vi "HOST.vi"() -> ()   [LabVIEW 2018]
uses:
  <vilib>/userdefined/High Color/nirio_resource_hc.ctl
  <instrlib>/niDCPower/nidcpower.llb/niDCPower Measurement Type.ctl
  <vilib>/FPGAPlugInAG/PXI-7953R/niLvFpga_Open_PXI-7953R.vi
  <vilib>/rvi/interface/common/dynamic/niFpgaDynamicAddResources.vi
  <vilib>/FPGAPlugInAG/Dynamic/niLvFpga_Reset_Dynamic.vi
  <vilib>/FPGAPlugInAG/Dynamic/niLvFpga_Run_Dynamic.vi
  <vilib>/Utility/error.llb/Error Cluster From Error Code.vi
  <vilib>/rvi/errors/niLvFpgaAdjustHostInterfaceError.vi
  <vilib>/rvi/interface/nirviOpenFPGA/nirviOpenFPGA.xnode
  FPGA Bitfiles/ILX751B20.008_FPGATarget_TARGET_7CPBKhOoNyI.lvbitx
  <vilib>/rvi/interface/nirviMethod/nirviMethod.xnode
  <vilib>/rvi/interface/nirviReadWriteControl/nirviReadWriteControl.xnode
  NiFpgaLv.dll
  <vilib>/rvi/interface/Simulation/niFpgaSimulationCallBeginRW.vi
  <vilib>/FPGAPlugInAG/Dynamic/niLvFpga_ReadFifo_Dynamic.vi
  <vilib>/rvi/errors/niLvFpgaMergeErrorWithErrorCode.vi
panel:
  in  "Какой шум на других каналах, мВ?":dbl
  in  "Кадр виден?":u32=50
  in  "3":refnum<k15>="PXI1Slot4" caption="1"
  in  "8191?":u16=8191
  out "DSNU, мВ":dbl
  out "PRNU, %":dbl
  out "|Vout|, мВ":dbl
  in  "Задержка, мкс":u16=7904
  in  "50?":u16=50
  in  "Светлый (T)\nТемный (F)":bool
  in  "Frames":path=path "C:/VPL/LabView_PRJ/ILX751B_20.008/FRAMES"
  in  "ПРИМЕЧАНИЕ":string
  out "Image":T1(plugin-control)
  out "Тнак, мс":dbl=10.0
  in  "Запись в FIFO":bool
  out "АЦП прошит!":bool
  in  "Какой канал?":enum16{"GREEN", "RED", "BLUE"}(ring)=enum."BLUE"
  in  "Усиление (до 6)_RED":u8=1
  in  "Усиление (до 6)_BLUE":u8=1
  in  "Усиление (до 6)_GREEN":u8=1
  in  "Смещение, до 300_BLUE":dbl
  in  "+/- BLUE":enum16{"-", "+"}(ring)=enum."+"
  in  "Смещение, до 300_RED":dbl
  in  "+/- RED":enum16{"-", "+"}(ring)=enum."+"
  in  "Смещение, до 300_GREEN":dbl
  in  "+/- GREEN":enum16{"-", "+"}(ring)=enum."+"
  in  "2/4 V":enum16{"2V", "4V"}(ring)=enum."4V"
  in  "3CH/1CH":enum16{"3CH", "1CH"}(ring)=enum."1CH"
  out "Configuration":bool[](array[boolean])
  in  "HIGH":u8=18
  in  "LOW":u8=8
  in  "CLK_1":u16=59
  in  "ROG_1":u16=20
  in  "ROG_2":u16=40
  in  "SHUT1":u16=120
  in  "CLK_2":u8=9
  in  "CLK_3":u8=20
  in  "20":u8=20
  in  "42000?":u16=42000
  in  "П_41789?":u16=41789
  in  "ADC_2":u8=13
  in  "ADC_1":u8=2
  in  "CDS2_2":u8=16
  in  "CDS2_1":u8=11
  in  "CDS1_2":u8=7
  in  "CDS1_1":u8=2
  in  "Линейки":bool
  in  "Направление бит":bool
  out "VDD2(5)":bool
  out "D_POW":bool
  out "VDD1(9)":bool
  out "A_POW":bool
  in  "VDD2(5)_selcur":dbl=0.019999999999999997 caption="current limit" format="%_6p"
  in  "D_POW_selcur":dbl=0.095 caption="current limit" format="%_6p"
  in  "VDD1(9)_selcur":dbl=0.02 caption="current limit" format="%_6p"
  in  "A_POW_selcur":dbl=0.095 caption="current limit" format="%_6p"
  out "VDD2(5)_char":dbl(graph)=-2.7174410869378702e-06
  out "D_POW_char":dbl(graph)=3.6139019911277516e-06
  in  "VDD2(5), V":dbl=5.0 caption="voltage level" format="%_6p"
  out "VDD2(5)_cur":dbl caption="measurement" format="%_6g"
  out "D_POW_cur":dbl caption="measurement" format="%_6g"
  in  "VDD2(5)_curlim":dbl=0.03 caption="current limit" format="%_6p"
  in  "D_POW_curlim":dbl=0.1 caption="current limit" format="%_6p"
  in  "D_POW, V":dbl=6.0 caption="voltage level" format="%_6p"
  out "VDD1(9)_char":dbl(graph)=-2.1008668383050173e-06
  out "A_POW_char":dbl(graph)=-8.364806008166422e-06
  in  "VDD1(9), V":dbl=9.0 caption="voltage level" format="%_6p"
  out "VDD1(9)_cur":dbl caption="measurement" format="%_6g"
  out "A_POW_cur":dbl caption="measurement" format="%_6g"
  in  "VDD1(9)_curlim":dbl=0.025 caption="current limit" format="%_6p"
  in  "A_POW_curlim":dbl=0.1 caption="current limit" format="%_6p"
  in  "A_POW, V":dbl=6.0 caption="voltage level" format="%_6p"
  in  "Запись кадра":bool
  in  "Прошить АЦП":bool
  in  "Стоп":bool
  in  "Питание":bool
  in  "1":refnum<k15>="PXI1Slot2"
  in  "2":refnum<k15>="PXI1Slot3" caption="1"
  in  "FPGA":T2="PXI1Slot6"
  in  "LOGS":path=path "C:/VPL/LabView_PRJ/ILX751B_20.008/LOGS"
  out "Номер образца":string="0"
  out "Температура":string="0"
  out "DATA":u16[][](array[numeric])=[[50262, 50314, 50369, 50314, 50358, 50311, 50219, 50342, 50335, 50313, 50333, 50279, 50363, 50343, 50274, 50276, 50233, 50283, 50311, 50287, 50326, 50286, 50307, 50313, 50307, 50331, 50315, 50337, 50306, 50335, 50319, 50301, 50336, 50227, 50277, 50229], [50350, 50364, 50285, 50278, 50292, 50197, 50322, 50306, 50283, 50316, 50366, 50335, 50361, 50305, 50282, 50331, 50289, 50304, 50280, 50343, 50359, 50302, 50322, 50214, 50283, 50259, 50363, 50351, 50343, 50321, 50257, 50285, 50351, 50343, 50338, 50332], [50366, 50361, 50275, 50313, 50304, 50293, 50288, 50317, 50370, 50362, 50234, 50266, 50286, 50291, 50335, 50393, 50273, 50357, 50309, 50337, 50280, 50288, 50318, 50296, 50332, 50300, 50286, 50237, 50266, 50342, 50300, 50253, 50340, 50319, 50339, 50302], [50354, 50256, 50301, 50345, 50299, 50339, 50302, 50346, 50308, 50371, 50355, 50325, 50269, 50290, 50285, 50295, 50330, 50336, 50273, 50328, 50381, 50309, 50322, 50368, 50264, 50312, 50320, 50313, 50312, 50334, 50268, 50322, 50334, 50286, 50261, 50358], [50287, 50325, 50343, 50290, 50297, 50249, 50310, 50231, 50393, 50382, 50314, 50281, 50335, 50394, 50319, 50265, 50294, 50289, 50347, 50253, 50336, 50295, 50322, 50299, 50378, 50258, 50375, 50333, 50303, 50337, 50319, 50319, 50298, 50267, 50314, 50295], [50353, 50353, 50335, 50237, 50317, 50296, 50234, 50359, 50320, 50320, 50278, 50331, 50287, 50292, 50318, 50341, 50385, 50311, 50376, 50379, 50338, 50414, 50297, 50260, 50227, 50299, 50319, 50396, 50380, 50305, 50335, 50281, 50362, 50368, 50336, 50293], [50306, 50281, 50350, 50290, 50282, 50309, 50310, 50345, 50257, 50309, 50334, 50377, 50244, 50252, 50260, 50349, 50408, 50298, 50304, 50320, 50314, 50316, 50265, 50294, 50400, 50263, 50304, 50272, 50319, 50392, 50327, 50280, 50360, 50255, 50358, 50361], [50350, 50246, 50307, 50293, 50282, 50315, 50263, 50291, 50402, 50315, 50351, 50325, 50369, 50243, 50347, 50363, 50304, 50328, 50247, 50311, 50333, 50430, 50262, 50343, 50369, 50284, 50307, 50319, 50305, 50258, 50334, 50339, 50319, 50380, 50365, 50363], [50349, 50329, 50280, 50304, 50335, 50280, 50314, 50306, 50298, 50357, 50316, 50381, 50295, 50289, 50218, 50298, 50346, 50225, 50386, 50297, 50333, 50311, 50310, 50235, 50280, 50290, 50309, 50275, 50289, 50386, 50273, 50300, 50357, 50360, 50305, 50350], [50332, 50310, 50312, 50284, 50303, 50332, 50307, 50290, 50276, 50337, 50376, 50371, 50329, 50360, 50328, 50316, 50329, 50346, 50292, 50326, 50338, 50284, 50331, 50256, 50333, 50351, 50274, 50375, 50312, 50302, 50347, 50301, 50341, 50276, 50235, 50295], [50368, 50274, 50286, 50317, 50311, 50276, 50267, 50303, 50282, 50301, 50318, 50259, 50361, 50309, 50320, 50255, 50223, 50330, 50380, 50312, 50369, 50261, 50323, 50266, 50374, 50210, 50374, 50289, 50329, 50331, 50301, 50281, 50270, 50310, 50367, 50268], [50304, 50349, 50357, 50309, 50320, 50276, 50360, 50358, 50320, 50316, 50280, 50238, 50371, 50312, 50236, 50334, 50295, 50391, 50334, 50300, 50341, 50353, 50305, 50233, 50234, 50266, 50322, 50294, 50306, 50397, 50267, 50307, 50365, 50369, 50336, 50331], [50309, 50374, 50308, 50336, 50307, 50284, 50361, 50352, 50378, 50343, 50340, 50308, 50268, 50279, 50363, 50340, 50314, 50294, 50299, 50325, 50276, 50301, 50383, 50309, 50320, 50314, 50266, 50391, 50338, 50232, 50405, 50285, 50299, 50281, 50352, 50288], [50324, 50243, 50342, 50322, 50352, 50352, 50305, 50253, 50309, 50250, 50270, 50266, 50292, 50292, 50351, 50309, 50317, 50312, 50360, 50335, 50310, 50304, 50262, 50340, 50305, 50309, 50320, 50321, 50328, 50282, 50334, 50304, 50300, 50320, 50305, 50313], [50326, 50354, 50306, 50316, 50338, 50313, 50369, 50327, 50318, 50357, 50354, 50312, 50363, 50327, 50338, 50381, 50312, 50319, 50261, 50309, 50318, 50354, 50349, 50340, 50356, 50325, 50291, 50232, 50350, 50346, 50276, 50383, 50290, 50281, 50281, 50342], [50361, 50273, 50328, 50306, 50307, 50246, 50290, 50388, 50343, 50389, 50305, 50283, 50336, 50403, 50288, 50346, 50371, 50282, 50355, 50334, 50297, 50351, 50387, 50371, 50289, 50292, 50321, 50269, 50295, 50356, 50238, 50360, 50346, 50359, 50314, 50301], [50252, 50301, 50331, 50337, 50242, 50286, 50276, 50311, 50302, 50325, 50333, 50308, 50329, 50327, 50344, 50354, 50316, 50272, 50257, 50354, 50361, 50344, 50372, 50284, 50301, 50326, 50348, 50334, 50366, 50302, 50291, 50302, 50285, 50349, 50279, 50285], [50295, 50324, 50312, 50371, 50300, 50301, 50322, 50338, 50385, 50358, 50374, 50369, 50315, 50364, 50239, 50389, 50322, 50323, 50272, 50333, 50322, 50343, 50313, 50268, 50362, 50359, 50315, 50302, 50358, 50329, 50299, 50295, 50263, 50367, 50354, 50277], [50285, 50253, 50337, 50323, 50334, 50348, 50350, 50292, 50307, 50305, 50262, 50413, 50304, 50307, 50286, 50313, 50318, 50406, 50369, 50319, 50306, 50385, 50329, 50396, 50247, 50377, 50372, 50334, 50322, 50381, 50364, 50304, 50325, 50317, 50330, 50190], [50336, 50338, 50322, 50295, 50419, 50350, 50295, 50371, 50329, 50321, 50293, 50299, 50347, 50374, 50348, 50310, 50349, 50397, 50395, 50242, 50273, 50312, 50298, 50291, 50343, 50312, 50338, 50295, 50327, 50323, 50416, 50285, 50281, 50289, 50289, 50308], [50348, 50318, 50252, 50326, 50350, 50324, 50311, 50284, 50307, 50361, 50328, 50345, 50294, 50315, 50312, 50390, 50336, 50273, 50349, 50286, 50363, 50346, 50322, 50316, 50335, 50349, 50311, 50275, 50298, 50273, 50344, 50269, 50287, 50349, 50376, 50296], [50346, 50375, 50300, 50310, 50332, 50321, 50281, 50344, 50327, 50344, 50314, 50296, 50264, 50303, 50292, 50249, 50272, 50352, 50341, 50286, 50350, 50288, 50264, 50288, 50339, 50331, 50304, 50306, 50316, 50303, 50273, 50326, 50293, 50312, 50371, 50314], [50323, 50330, 50320, 50367, 50295, 50329, 50297, 50278, 50345, 50341, 50284, 50252, 50343, 50350, 50360, 50332, 50276, 50305, 50345, 50342, 50314, 50376, 50420, 50322, 50313, 50363, 50318, 50338, 50333, 50290, 50335, 50263, 50301, 50286, 50337, 50249], [50343, 50348, 50377, 50338, 50382, 50269, 50308, 50370, 50305, 50383, 50350, 50392, 50367, 50304, 50281, 50327, 50286, 50313, 50308, 50270, 50333, 50319, 50326, 50282, 50395, 50342, 50297, 50331, 50297, 50323, 50275, 50276, 50323, 50278, 50279, 50321], [50230, 50351, 50349, 50291, 50304, 50283, 50315, 50264, 50387, 50292, 50319, 50259, 50376, 50275, 50388, 50293, 50343, 50254, 50299, 50334, 50276, 50381, 50315, 50347, 50303, 50278, 50376, 50293, 50367, 50287, 50311, 50340, 50288, 50319, 50375, 50299], [50304, 50338, 50255, 50333, 50353, 50298, 50321, 50241, 50274, 50296, 50317, 50350, 50284, 50385, 50270, 50276, 50349, 50228, 50340, 50267, 50376, 50352, 50328, 50286, 50267, 50386, 50324, 50342, 50331, 50339, 50331, 50346, 50355, 50319, 50271, 50291], [50315, 50259, 50331, 50329, 50311, 50329, 50347, 50403, 50324, 50381, 50316, 50273, 50285, 50338, 50298, 50312, 50326, 50298, 50307, 50387, 50362, 50315, 50299, 50383, 50327, 50393, 50323, 50285, 50357, 50387, 50270, 50325, 50308, 50338, 50231, 50285], [50384, 50350, 50363, 50391, 50340, 50290, 50319, 50355, 50291, 50418, 50347, 50265, 50239, 50265, 50343, 50343, 50400, 50315, 50292, 50367, 50345, 50326, 50293, 50318, 50345, 50256, 50297, 50262, 50363, 50380, 50330, 50346, 50331, 50429, 50274, 50273], [50329, 50359, 50330, 50399, 50308, 50368, 50289, 50321, 50333, 50340, 50276, 50410, 50324, 50324, 50356, 50370, 50327, 50278, 50340, 50392, 50355, 50329, 50375, 50282, 50324, 50353, 50288, 50345, 50281, 50350, 50254, 50322, 50266, 50288, 50267, 50287], [50397, 50341, 50356, 50357, 50321, 50300, 50278, 50294, 50284, 50374, 50242, 50349, 50325, 50326, 50243, 50309, 50404, 50316, 50279, 50313, 50314, 50334, 50274, 50285, 50328, 50315, 50279, 50271, 50340, 50340, 50287, 50351, 50355, 50322, 50284, 50339], [50345, 50387, 50385, 50288, 50353, 50322, 50341, 50374, 50340, 50316, 50369, 50362, 50341, 50276, 50336, 50288, 50347, 50316, 50340, 50258, 50320, 50319, 50292, 50392, 50381, 50374, 50329, 50280, 50310, 50356, 50373, 50386, 50344, 50265, 50250, 50334], [50321, 50238, 50340, 50279, 50339, 50338, 50323, 50336, 50357, 50311, 50365, 50345, 50274, 50350, 50395, 50322, 50330, 50347, 50291, 50291, 50299, 50361, 50255, 50331, 50301, 50305, 50274, 50297, 50363, 50392, 50252, 50391, 50286, 50387, 50278, 50300], [50217, 50371, 50307, 50339, 50290, 50314, 50315, 50337, 50319, 50307, 50239, 50341, 50350, 50283, 50349, 50361, 50338, 50295, 50305, 50344, 50318, 50265, 50273, 50350, 50284, 50361, 50226, 50334, 50331, 50316, 50314, 50319, 50297, 50261, 50266, 50315], [50279, 50360, 50294, 50297, 50343, 50325, 50286, 50335, 50258, 50295, 50374, 50267, 50359, 50313, 50265, 50281, 50287, 50343, 50338, 50356, 50330, 50309, 50297, 50345, 50330, 50329, 50320, 50320, 50340, 50311, 50264, 50258, 50334, 50294, 50287, 50320], [50297, 50313, 50389, 50289, 50356, 50348, 50342, 50368, 50390, 50300, 50328, 50251, 50290, 50217, 50338, 50416, 50363, 50333, 50326, 50301, 50270, 50301, 50264, 50365, 50290, 50299, 50302, 50326, 50304, 50303, 50289, 50269, 50319, 50290, 50293, 50322], [50294, 50349, 50301, 50344, 50301, 50333, 50344, 50296, 50326, 50380, 50368, 50268, 50284, 50287, 50296, 50302, 50336, 50278, 50299, 50352, 50311, 50302, 50275, 50315, 50360, 50293, 50355, 50299, 50323, 50298, 50356, 50279, 50343, 50337, 50251, 50336], [50247, 50377, 50328, 50357, 50314, 50287, 50326, 50310, 50324, 50323, 50325, 50313, 50327, 50304, 50329, 50250, 50348, 50455, 50386, 50310, 50383, 50312, 50349, 50233, 50295, 50397, 50284, 50320, 50260, 50291, 50328, 50278, 50336, 50262, 50259, 50306], [50359, 50342, 50327, 50305, 50335, 50317, 50367, 50285, 50340, 50357, 50344, 50287, 50346, 50348, 50290, 50304, 50343, 50297, 50328, 50381, 50298, 50265, 50406, 50262, 50350, 50269, 50206, 50385, 50325, 50265, 50298, 50293, 50374, 50284, 50352, 50335], [50342, 50353, 50288, 50360, 50419, 50337, 50312, 50326, 50324, 50359, 50356, 50300, 50215, 50284, 50335, 50312, 50328, 50287, 50316, 50281, 50298, 50302, 50289, 50322, 50368, 50289, 50333, 50250, 50291, 50346, 50270, 50304, 50321, 50363, 50343, 50331], [50352, 50280, 50263, 50251, 50331, 50290, 50298, 50329, 50399, 50351, 50337, 50287, 50304, 50329, 50381, 50376, 50343, 50284, 50320, 50242, 50308, 50273, 50288, 50316, 50379, 50336, 50260, 50350, 50378, 50349, 50290, 50334, 50275, 50291, 50376, 50283], [50377, 50367, 50281, 50214, 50311, 50318, 50299, 50270, 50249, 50259, 50321, 50371, 50315, 50290, 50285, 50286, 50255, 50359, 50385, 50386, 50221, 50283, 50329, 50352, 50261, 50308, 50291, 50272, 50294, 50354, 50296, 50299, 50288, 50297, 50275, 50292], [50321, 50326, 50282, 50349, 50268, 50298, 50309, 50365, 50344, 50278, 50341, 50362, 50340, 50230, 50289, 50230, 50327, 50354, 50325, 50358, 50403, 50299, 50351, 50286, 50269, 50319, 50317, 50279, 50235, 50254, 50369, 50348, 50367, 50341, 50277, 50288], [50332, 50357, 50278, 50248, 50312, 50294, 50258, 50305, 50374, 50310, 50361, 50311, 50304, 50341, 50247, 50336, 50337, 50320, 50350, 50351, 50310, 50320, 50258, 50287, 50285, 50347, 50402, 50355, 50293, 50294, 50303, 50367, 50295, 50294, 50329, 50303], [50279, 50371, 50307, 50324, 50277, 50281, 50353, 50317, 50318, 50254, 50314, 50422, 50282, 50269, 50277, 50303, 50355, 50297, 50286, 50318, 50297, 50311, 50370, 50221, 50315, 50356, 50313, 50309, 50254, 50291, 50308, 50240, 50252, 50371, 50403, 50380], [50296, 50318, 50429, 50315, 50282, 50342, 50311, 50282, 50247, 50303, 50323, 50329, 50299, 50389, 50305, 50253, 50294, 50473, 50292, 50316, 50336, 50411, 50408, 50318, 50254, 50356, 50375, 50344, 50355, 50207, 50306, 50327, 50346, 50289, 50303, 50265], [50363, 50305, 50264, 50319, 50350, 50281, 50322, 50336, 50355, 50293, 50298, 50335, 50306, 50329, 50272, 50319, 50333, 50251, 50390, 50284, 50327, 50276, 50301, 50321, 50338, 50295, 50352, 50354, 50386, 50361, 50257, 50276, 50313, 50327, 50352, 50264], [50260, 50306, 50291, 50288, 50350, 50326, 50331, 50273, 50306, 50313, 50309, 50301, 50326, 50347, 50302, 50382, 50372, 50269, 50347, 50289, 50299, 50366, 50324, 50345, 50344, 50295, 50287, 50270, 50352, 50300, 50271, 50301, 50287, 50360, 50264, 50345], [50316, 50327, 50336, 50252, 50314, 50342, 50357, 50370, 50330, 50245, 50305, 50260, 50349, 50353, 50288, 50296, 50286, 50282, 50276, 50284, 50358, 50245, 50323, 50312, 50298, 50303, 50334, 50301, 50338, 50359, 50379, 50299, 50300, 50325, 50343, 50263], [50287, 50306, 50332, 50297, 50215, 50337, 50371, 50298, 50288, 50337, 50324, 50279, 50309, 50296, 50254, 50354, 50333, 50334, 50284, 50405, 50367, 50340, 50281, 50342, 50380, 50341, 50346, 50278, 50261, 50274, 50358, 50281, 50385, 50296, 50275, 50327], [50314, 50340, 50342, 50367, 50309, 50319, 50338, 50379, 50283, 50366, 50347, 50367, 50387, 50229, 50327, 50299, 50243, 50327, 50328, 50345, 50309, 50365, 50321, 50308, 50294, 50306, 50234, 50310, 50306, 50305, 50351, 50403, 50319, 50279, 50270, 50321], [50295, 50311, 50369, 50283, 50256, 50277, 50329, 50350, 50267, 50314, 50384, 50340, 50413, 50363, 50295, 50252, 50246, 50358, 50337, 50355, 50258, 50313, 50327, 50298, 50319, 50399, 50312, 50391, 50305, 50321, 50301, 50336, 50309, 50312, 50300, 50356], [50376, 50314, 50302, 50290, 50314, 50346, 50351, 50319, 50271, 50279, 50305, 50351, 50281, 50363, 50385, 50350, 50357, 50318, 50279, 50330, 50307, 50314, 50335, 50329, 50345, 50317, 50295, 50371, 50258, 50330, 50374, 50239, 50353, 50387, 50329, 50325], [50285, 50280, 50265, 50316, 50314, 50264, 50258, 50262, 50350, 50381, 50336, 50281, 50345, 50305, 50252, 50358, 50318, 50314, 50340, 50334, 50265, 50331, 50305, 50394, 50319, 50374, 50381, 50286, 50349, 50335, 50353, 50380, 50237, 50324, 50283, 50374], [50318, 50292, 50336, 50265, 50301, 50291, 50300, 50336, 50292, 50308, 50363, 50352, 50284, 50342, 50272, 50349, 50476, 50358, 50261, 50350, 50336, 50400, 50421, 50284, 50345, 50320, 50278, 50344, 50338, 50366, 50272, 50323, 50316, 50339, 50371, 50198], [50359, 50322, 50413, 50297, 50295, 50361, 50233, 50330, 50260, 50259, 50350, 50374, 50293, 50306, 50325, 50331, 50295, 50286, 50277, 50360, 50331, 50405, 50243, 50326, 50320, 50333, 50306, 50367, 50343, 50346, 50294, 50309, 50319, 50361, 50361, 50315], [50312, 50309, 50306, 50336, 50269, 50332, 50258, 50295, 50304, 50366, 50386, 50385, 50215, 50292, 50281, 50355, 50290, 50333, 50282, 50216, 50323, 50287, 50350, 50355, 50338, 50275, 50315, 50353, 50325, 50317, 50307, 50399, 50302, 50370, 50346, 50269], [50239, 50355, 50305, 50347, 50338, 50337, 50257, 50334, 50253, 50315, 50306, 50374, 50387, 50344, 50365, 50329, 50317, 50357, 50332, 50338, 50350, 50308, 50258, 50306, 50291, 50335, 50362, 50323, 50325, 50347, 50293, 50367, 0, 0, 0, 50266], [50265, 50281, 50002, 50308, 50309, 50282, 50304, 50313, 50318, 50294, 50341, 50296, 50342, 50319, 50361, 50354, 50328, 50217, 50303, 50266, 50393, 50366, 50374, 50243, 50307, 50246, 50331, 50271, 50223, 50271, 50323, 50293, 50207, 50289, 50339, 0]]
  # "ПРЕДЛАГАЮ БРАТЬ ЗА НАСЫЩЕНИЕ МАКСИМАЛЬНО ДОСТИЖИМОЕ ЗНАЧЕНИЕ"
  # "7904 и 120"
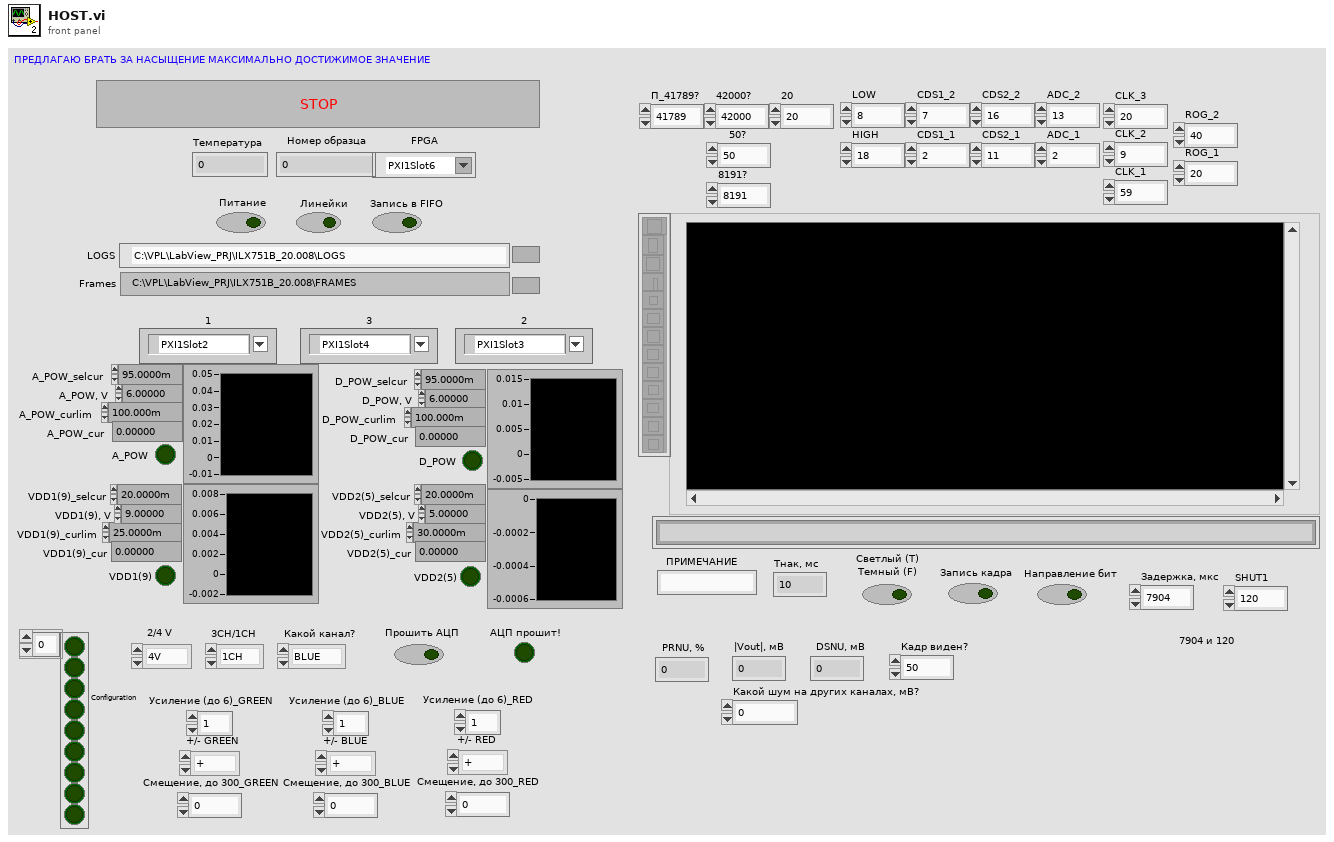
[diagram p1: front panel]
types:
  T1 = typedef "IMAQ Image.ctl" = refnum<image>
  T2 = typedef "nirio_resource_hc.ctl" = tag
  T3 = enum16{"open", "replace", "create", "open or create", "replace or create", "replace or create with confirmation"}
  T4 = enum16{"Configuration", "MUX", "RED PGA", "GREEN PGA", "BLUE PGA", "RED OFF", "GREEN OFF", "BLUE OFF"}
  T5 = typedef "Image Type" = u32
  T6 = typedef "niDCPower Measurement Type.ctl" = i32
  T7 = cluster{"Global Rectangle":i32[], "Contours":cluster{"Contour Type":u32, "ROI Type":u32, "Points":i32[]}[]}
  T8 = cluster{"Contour Type":u32, "ROI Type":u32, "Points":i32[]}[]
  T9 = cluster{"Contour Type":u32, "ROI Type":u32, "Points":i32[]}
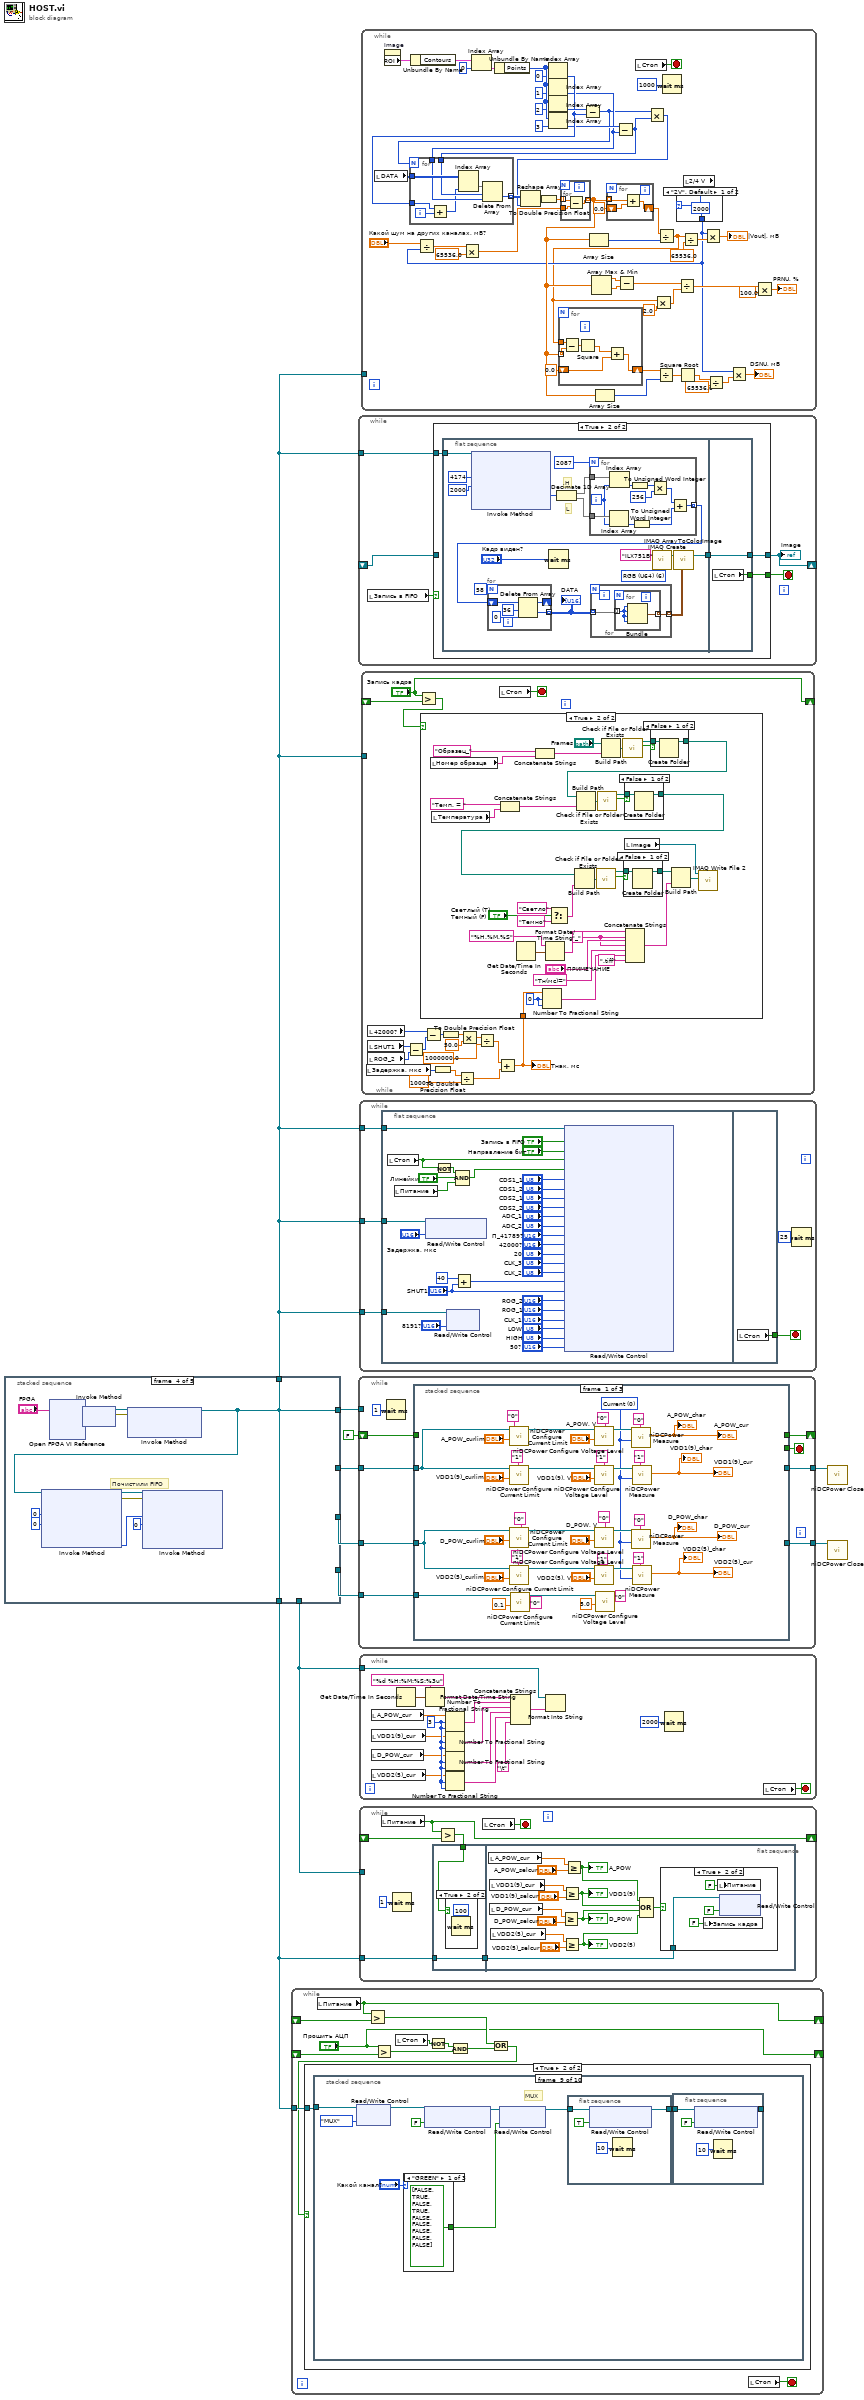
[diagram p0: block diagram]
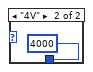
[diagram p2: hidden frame]
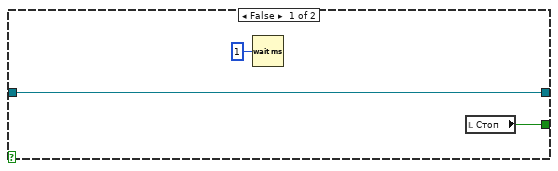
[diagram p3: hidden frame]
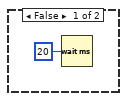
[diagram p4: hidden frame]
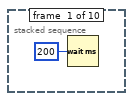
[diagram p5: hidden frame]
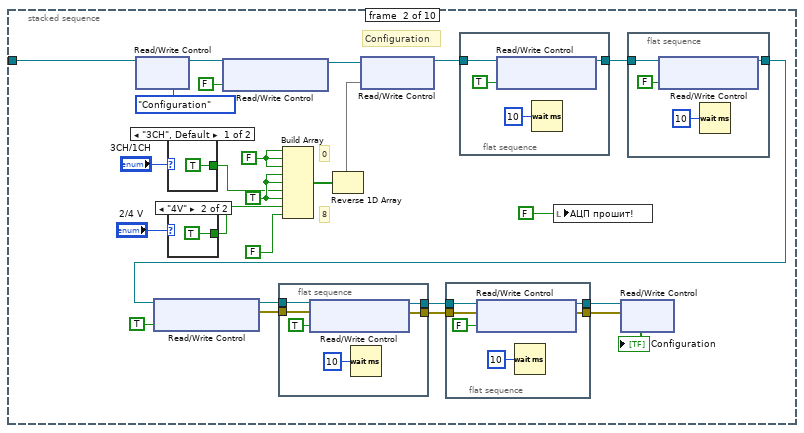
[diagram p6: hidden frame]
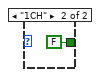
[diagram p7: hidden frame]
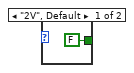
[diagram p8: hidden frame]
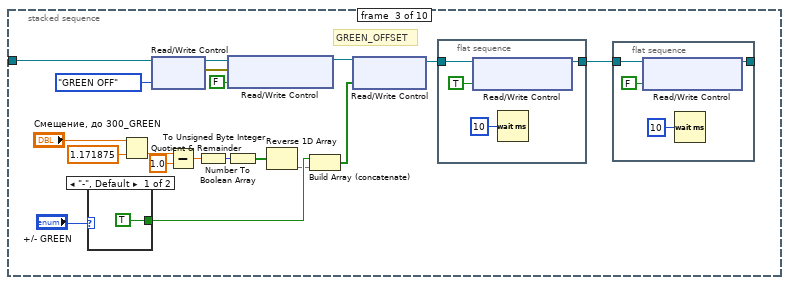
[diagram p9: hidden frame]
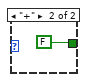
[diagram p10: hidden frame]
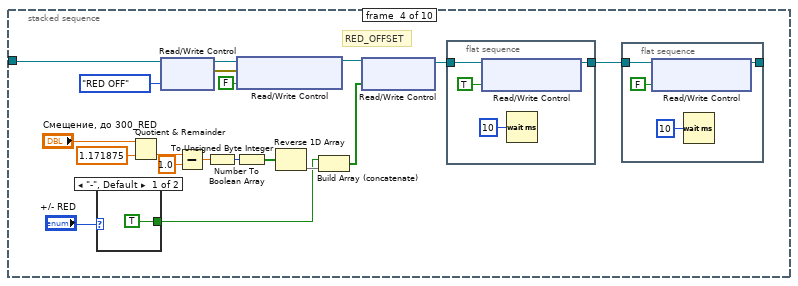
[diagram p11: hidden frame]
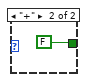
[diagram p12: hidden frame]
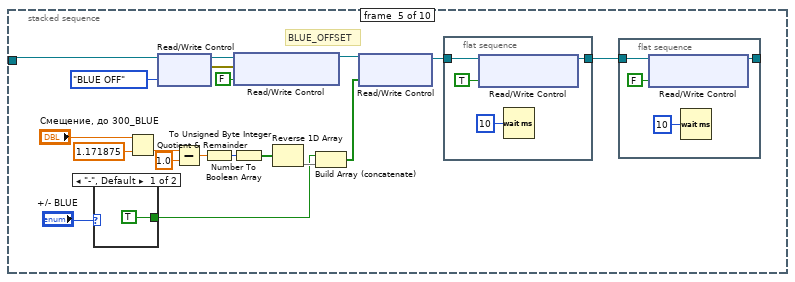
[diagram p13: hidden frame]
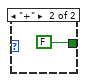
[diagram p14: hidden frame]
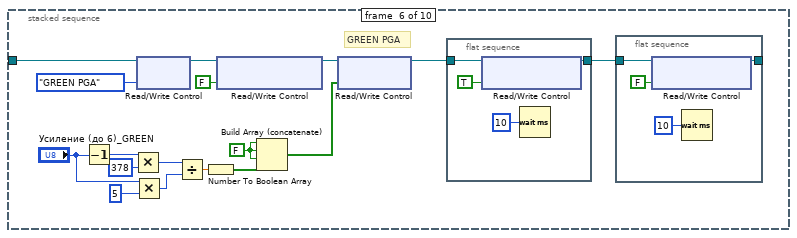
[diagram p15: hidden frame]
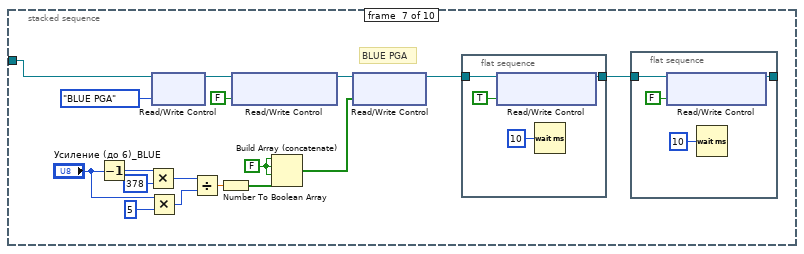
[diagram p16: hidden frame]
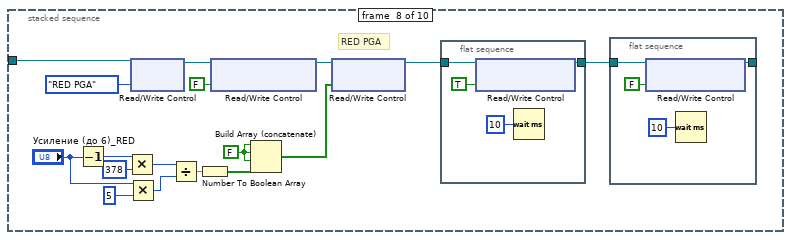
[diagram p17: hidden frame]
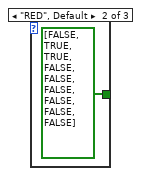
[diagram p18: hidden frame]
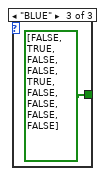
[diagram p19: hidden frame]
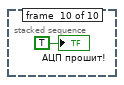
[diagram p20: hidden frame]
diagram:
  n1 = stacked-sequence {
    tunnel: [_ _ _ w61 _] -> w8
    tunnel: [_ _ _ _ w82] -> w10
    tunnel: [_ _ _ _ w81] -> w9
    tunnel: [_ _ _ w61 _] -> w1
    tunnel: [_ _ _ w61 _] -> w3
    tunnel: [_ _ w29 _ _] -> w4
    tunnel: [_ _ _ _ w73] -> w2
    frame #0 {
      n2 = call "Begin.vi"() -> ("Температура 2"=→"Температура":string, "Номер образца 2"=→"Номер образца":string)  [unwired: 10 in]
    }
    frame #1 {
      # "Обнуление всего"
      n3 = local write "Прошить АЦП"(FALSE ("Прошить АЦП")) -> ()
      n4 = local write "Запись кадра"(FALSE ("FRAME!")) -> ()
      n5 = local write "Питание"(FALSE ("Питание")) -> ()
      n6 = local write "Стоп"(FALSE ("Стоп")) -> ()
      n7 = local write "VDD1(9)"(FALSE ("VDD1(9)")) -> ()
      n8 = local write "VDD2(5)"(FALSE ("VDD2(5)")) -> ()
      n9 = local write "A_POW"(FALSE ("A_POW")) -> ()
      n10 = local write "D_POW"(FALSE ("D_POW")) -> ()
    }
    frame #2 {
      w22 = "\t"
      n11 = local read "Номер образца"() -> (w50:string)
      n12 = Build Path(base path="LOGS", name or relative path=w50) -> (appended path=w47:path)
      n13 = Get Date/Time In Seconds() -> (seconds since 1Jan1904=w44:timestamp)
      n14 = call <vilib>:"Check if File or Folder Exists.vi"("path"=w47) -> ("file or folder exists?"=w48:bool, "dup path"=w49:path)  [unwired: 8 in, 1 out]
      n15 = local read "Температура"() -> (w24:string)
      n16 = Format Date/Time String(time format string (%c)="%d %H.%M.%S", seconds (now)=w44) -> (date/time string=w42:string)  [unwired: 1 in]
      n17 = case shown="False" w48 {
        tunnel: w49 -> [w59 w60]
        tunnel: [w58 w60] -> w25
        frame False {
          n18 = Create Folder(path (use dialog)=w59) -> (created path=w58:path)  [unwired: 2 in, 2 out]
        }
        frame True {
        }
      }
      n19 = Concatenate Strings(w42, ".xls" ("string")) -> (w41:string)
      n20 = Build Path(base path=w25, name or relative path=w24) -> (appended path=w28:path)
      n21 = call <vilib>:"Check if File or Folder Exists.vi"("path"=w28) -> ("file or folder exists?"=w27:bool, "dup path"=w26:path)  [unwired: 8 in, 1 out]
      n22 = case shown="False" w27 {
        tunnel: w26 -> [w52 w53]
        tunnel: [w51 w53] -> w23
        frame False {
          n23 = Create Folder(path (use dialog)=w52) -> (created path=w51:path)  [unwired: 2 in, 2 out]
        }
        frame True {
        }
      }
      n24 = Build Path(base path=w23, name or relative path=w41) -> (appended path=w43:path)
      n25 = Open/Create/Replace File(file path (use dialog)=w43, operation (0:open)=T3."open or create", access (0:read/write)=enum16{"read/write", "read-only", "write-only"}."read/write") -> (refnum out=w45:refnum<file>)  [unwired: 3 in, 2 out]
      n26 = case shown="True" TRUE {
        tunnel: w45 -> [w54 w57]
        tunnel: [w54 w55] -> w40
        frame False {
        }
        frame True {
          n27 = Set File Position(refnum=w57, from (0:start)=enum16{"start", "end", "current"}."end") -> (refnum out=w55:refnum<file>)  [unwired: 2 in, 1 out]
        }
      }
      n28 = Format Into String(initial string=w40, "Time" ("input 1"), w22, "A_POW_cur", w22, "VDD1_cur", w22, "D_POW_cur", w22, "VDD2_cur", "\r\n") -> (resulting string=w29:refnum<file>)  [unwired: 2 in, 1 out]
    }
    frame #3 {
      # "Почистили FIFO"
      n29 = xnode "Open FPGA VI Reference"("resource name"="FPGA") -> ("FPGA VI Reference Out"=w69:refnum<k20>, "error out"=w71:errorcluster)  [unwired: 1 in]
      n30 = xnode "Invoke Method"("FPGA VI Reference In"=w69, "error in"=w71) -> ("FPGA VI Reference Out"=w72:refnum<k20>, "error out"=w70:errorcluster)
      n31 = xnode "Invoke Method"("FPGA VI Reference In"=w72, "error in"=w70) -> ("FPGA VI Reference Out"=w61:refnum<k20>)  [unwired: 1 in, 1 out]
      n32 = xnode "Invoke Method"("FPGA VI Reference In"=w61, "Number of Elements"=u32 0, "Timeout (ms)"=0) -> ("FPGA VI Reference Out"=w67:refnum<k20>, "error out"=w66:errorcluster, "Elements Remaining"=w65:u32)  [unwired: 1 in, 1 out]
      n33 = xnode "Invoke Method"("FPGA VI Reference In"=w67, "error in"=w66, "Number of Elements"=w65, "Timeout (ms)"=0) -> ()  [unwired: 4 out]
    }
    frame #4 {
      n34 = call <instrlib>:"niDCPower Initialize.vi"("resource name"="3") -> ("error out"=w76:errorcluster, "instrument handle out"=w77:refnum<k15>)  [unwired: 3 in, 6 out]
      n35 = call <instrlib>:"niDCPower Initialize.vi"("resource name"="2") -> ("error out"=w85:errorcluster, "instrument handle out"=w83:refnum<k15>)  [unwired: 3 in, 6 out]
      n36 = call <instrlib>:"niDCPower Initialize.vi"("resource name"="1") -> ("error out"=w86:errorcluster, "instrument handle out"=w84:refnum<k15>)  [unwired: 3 in, 6 out]
      n37 = call <instrlib>:"niDCPower Configure Voltage Level.vi"("error in (no error)"=w76, "voltage level"=0.0, "channel name"="0", "instrument handle"=w77) -> ("instrument handle out"=w73:refnum<k15>)  [unwired: 6 in, 1 out]
      n38 = call <instrlib>:"niDCPower Configure Voltage Level.vi"("error in (no error)"=w85, "voltage level"=0.0, "channel name"="0,1", "instrument handle"=w83) -> ("instrument handle out"=w81:refnum<k15>)  [unwired: 6 in, 1 out]
      n39 = call <instrlib>:"niDCPower Configure Voltage Level.vi"("error in (no error)"=w86, "voltage level"=0.0, "channel name"="0,1", "instrument handle"=w84) -> ("instrument handle out"=w82:refnum<k15>)  [unwired: 6 in, 1 out]
    }
  }
  n40 = while {
    tunnel: w3 -> [w101]
    shift-right: ["Прошить АЦП"] -> _
    shift-left: _ -> [w100]
    shift-right: [w96] -> _
    shift-left: _ -> [w97]
    stop <- w102 stop-if-true
    n41 = local read "Питание"() -> (w96:bool)
    n42 = Greater?(x=w96, y=w97) -> (0:w95:bool)
    n43 = Greater?(x="Прошить АЦП", y=w100) -> (0:w99:bool)
    n44 = local read "Стоп"() -> (w92:bool)
    n45 = Not(x=w92) -> (.not. x?=w91:bool)
    n46 = And(x=w91, y=w99) -> (x .and. y?=w98:bool)
    n47 = Or(x=w95, y=w98) -> (x .or. y?=w94:bool)
    n48 = case shown="True" w94 {
      tunnel: w101 -> [_ w104]
      frame False {
        n49 = Wait (ms)(milliseconds to wait=u32 20) -> ()  [unwired: 1 out]
      }
      frame True {
        n50 = stacked-sequence {
          tunnel: w104 -> [_ w131 w171 w185 w214 w258 w268 w293 w326 _]
          frame #0 {
            n51 = Wait (ms)(milliseconds to wait=u32 200) -> ()  [unwired: 1 out]
          }
          frame #1 {
            w127 = TRUE ("element")
            w128 = FALSE
            # "8"
            # "0"
            # "Configuration"
            n52 = xnode "Read/Write Control"("FPGA VI Reference In"=w131, "Enum"=T4."Configuration") -> ("FPGA VI Reference Out"=w118:refnum<k20>)  [unwired: 1 in, 1 out]
            n53 = xnode "Read/Write Control"("FPGA VI Reference In"=w108, "Read(T)/Write(F)"=TRUE) -> ("FPGA VI Reference Out"=w114:refnum<k20>, "error out"=w113:errorcluster)  [unwired: 1 in]
            n54 = case shown="\"3CH\", Default" "3CH/1CH" {
              tunnel: [TRUE FALSE] -> w126
              frame "3CH", Default {
              }
              frame "1CH" {
              }
            }
            n55 = case shown="\"4V\"" "2/4 V" {
              tunnel: [FALSE TRUE] -> w124
              frame "2V", Default {
              }
              frame "4V" {
              }
            }
            n56 = xnode "Read/Write Control"("FPGA VI Reference In"=w118, "Read(T)/Write(F)"=FALSE) -> ("FPGA VI Reference Out"=w116:refnum<k20>)  [unwired: 1 in, 1 out]
            n57 = flat-sequence {
              tunnel: w114 -> [w143]
              tunnel: w113 -> [w142]
              tunnel: [w141] -> w112
              tunnel: [w140] -> w111
              frame #0 {
                n58 = xnode "Read/Write Control"("FPGA VI Reference In"=w143, "error in"=w142, "Конфигурация"=TRUE) -> ("FPGA VI Reference Out"=w141:refnum<k20>, "error out"=w140:errorcluster)
                n59 = Wait (ms)(milliseconds to wait=u32 10) -> ()  [unwired: 1 out]
              }
            }
            n60 = Build Array(w128, w128, w128, w127, w127, w126, w127, w124, FALSE) -> (w129:bool[])
            n61 = Reverse 1D Array(array=w129) -> (reversed array=w121:bool[])
            n62 = xnode "Read/Write Control"("FPGA VI Reference In"=w116, "Write Data"=w121) -> ("FPGA VI Reference Out"=w120:refnum<k20>)  [unwired: 1 in, 1 out]
            n63 = flat-sequence {
              tunnel: w112 -> [w137]
              tunnel: w111 -> [w136]
              tunnel: [w134] -> w110
              tunnel: [w133] -> w109
              frame #0 {
                n64 = xnode "Read/Write Control"("FPGA VI Reference In"=w137, "error in"=w136, "Конфигурация"=FALSE) -> ("FPGA VI Reference Out"=w134:refnum<k20>, "error out"=w133:errorcluster)
                n65 = Wait (ms)(milliseconds to wait=u32 10) -> ()  [unwired: 1 out]
              }
            }
            n66 = flat-sequence {
              tunnel: w120 -> [w151]
              tunnel: [w149] -> w119
              frame #0 {
                n67 = xnode "Read/Write Control"("FPGA VI Reference In"=w151, "Конфигурация"=TRUE) -> ("FPGA VI Reference Out"=w149:refnum<k20>)  [unwired: 1 in, 1 out]
                n68 = Wait (ms)(milliseconds to wait=u32 10) -> ()  [unwired: 1 out]
              }
            }
            n69 = local write "АЦП прошит!"(FALSE ("АЦП прошит!")) -> ()
            n70 = xnode "Read/Write Control"("FPGA VI Reference In"=w110, "error in"=w109) -> ("READ"=→"Configuration":bool[])  [unwired: 2 out]
            n71 = flat-sequence {
              tunnel: w119 -> [w147]
              tunnel: [w145] -> w108
              frame #0 {
                n72 = xnode "Read/Write Control"("FPGA VI Reference In"=w147, "Конфигурация"=FALSE) -> ("FPGA VI Reference Out"=w145:refnum<k20>)  [unwired: 1 in, 1 out]
                n73 = Wait (ms)(milliseconds to wait=u32 10) -> ()  [unwired: 1 out]
              }
            }
          }
          frame #2 {
            # "GREEN_OFFSET"
            n74 = case shown="\"-\", Default" "+/- GREEN" {
              tunnel: [TRUE FALSE] -> w158
              frame "-", Default {
              }
              frame "+" {
              }
            }
            n75 = Quotient & Remainder(x="Смещение, до 300_GREEN", y=1.171875) -> (floor(x/y)=w163:dbl)  [unwired: 1 out]
            n76 = xnode "Read/Write Control"("FPGA VI Reference In"=w171, "Enum"=T4."GREEN OFF" ("OFFSET")) -> ("FPGA VI Reference Out"=w170:refnum<k20>, "error out"=w169:errorcluster)  [unwired: 1 in]
            n77 = Subtract(x=w163, y=1.0) -> (x-y=w160:dbl)
            n78 = To Unsigned Byte Integer(number=w160) -> (unsigned 8bit integer=w159:u8)
            n79 = xnode "Read/Write Control"("FPGA VI Reference In"=w170, "error in"=w169, "Read(T)/Write(F)"=FALSE) -> ("FPGA VI Reference Out"=w168:refnum<k20>)  [unwired: 1 out]
            n80 = Number To Boolean Array(number=w159) -> (Boolean array=w157:bool[])
            n81 = Reverse 1D Array(array=w157) -> (reversed array=w156:bool[])
            n82 = Build Array (concatenate)(w158, w156) -> (w161:bool[])
            n83 = xnode "Read/Write Control"("FPGA VI Reference In"=w168, "Write Data"=w161) -> ("FPGA VI Reference Out"=w173:refnum<k20>)  [unwired: 1 in, 1 out]
            n84 = flat-sequence {
              tunnel: w173 -> [w184]
              tunnel: [w182] -> w172
              frame #0 {
                n85 = xnode "Read/Write Control"("FPGA VI Reference In"=w184, "Конфигурация"=TRUE) -> ("FPGA VI Reference Out"=w182:refnum<k20>)  [unwired: 1 in, 1 out]
                n86 = Wait (ms)(milliseconds to wait=u32 10) -> ()  [unwired: 1 out]
              }
            }
            n87 = flat-sequence {
              tunnel: w172 -> [w180]
              tunnel: [w178] -> _
              frame #0 {
                n88 = xnode "Read/Write Control"("FPGA VI Reference In"=w180, "Конфигурация"=FALSE) -> ("FPGA VI Reference Out"=w178:refnum<k20>)  [unwired: 1 in, 1 out]
                n89 = Wait (ms)(milliseconds to wait=u32 10) -> ()  [unwired: 1 out]
              }
            }
          }
          frame #3 {
            # "RED_OFFSET"
            n90 = case shown="\"-\", Default" "+/- RED" {
              tunnel: [TRUE FALSE] -> w201
              frame "-", Default {
              }
              frame "+" {
              }
            }
            n91 = Quotient & Remainder(x="Смещение, до 300_RED", y=1.171875) -> (floor(x/y)=w196:dbl)  [unwired: 1 out]
            n92 = xnode "Read/Write Control"("FPGA VI Reference In"=w185, "Enum"=T4."RED OFF" ("OFFSET")) -> ("FPGA VI Reference Out"=w192:refnum<k20>, "error out"=w193:errorcluster)  [unwired: 1 in]
            n93 = Subtract(x=w196, y=1.0) -> (x-y=w199:dbl)
            n94 = To Unsigned Byte Integer(number=w199) -> (unsigned 8bit integer=w200:u8)
            n95 = xnode "Read/Write Control"("FPGA VI Reference In"=w192, "error in"=w193, "Read(T)/Write(F)"=FALSE) -> ("FPGA VI Reference Out"=w194:refnum<k20>)  [unwired: 1 out]
            n96 = Number To Boolean Array(number=w200) -> (Boolean array=w202:bool[])
            n97 = Reverse 1D Array(array=w202) -> (reversed array=w203:bool[])
            n98 = Build Array (concatenate)(w201, w203) -> (w198:bool[])
            n99 = xnode "Read/Write Control"("FPGA VI Reference In"=w194, "Write Data"=w198) -> ("FPGA VI Reference Out"=w190:refnum<k20>)  [unwired: 1 in, 1 out]
            n100 = flat-sequence {
              tunnel: w190 -> [w213]
              tunnel: [w211] -> w191
              frame #0 {
                n101 = xnode "Read/Write Control"("FPGA VI Reference In"=w213, "Конфигурация"=TRUE) -> ("FPGA VI Reference Out"=w211:refnum<k20>)  [unwired: 1 in, 1 out]
                n102 = Wait (ms)(milliseconds to wait=u32 10) -> ()  [unwired: 1 out]
              }
            }
            n103 = flat-sequence {
              tunnel: w191 -> [w209]
              tunnel: [w207] -> _
              frame #0 {
                n104 = xnode "Read/Write Control"("FPGA VI Reference In"=w209, "Конфигурация"=FALSE) -> ("FPGA VI Reference Out"=w207:refnum<k20>)  [unwired: 1 in, 1 out]
                n105 = Wait (ms)(milliseconds to wait=u32 10) -> ()  [unwired: 1 out]
              }
            }
          }
          frame #4 {
            # "BLUE_OFFSET"
            n106 = case shown="\"-\", Default" "+/- BLUE" {
              tunnel: [TRUE FALSE] -> w230
              frame "-", Default {
              }
              frame "+" {
              }
            }
            n107 = Quotient & Remainder(x="Смещение, до 300_BLUE", y=1.171875) -> (floor(x/y)=w225:dbl)  [unwired: 1 out]
            n108 = xnode "Read/Write Control"("FPGA VI Reference In"=w214, "Enum"=T4."BLUE OFF" ("OFFSET")) -> ("FPGA VI Reference Out"=w221:refnum<k20>, "error out"=w222:errorcluster)  [unwired: 1 in]
            n109 = Subtract(x=w225, y=1.0) -> (x-y=w228:dbl)
            n110 = To Unsigned Byte Integer(number=w228) -> (unsigned 8bit integer=w229:u8)
            n111 = xnode "Read/Write Control"("FPGA VI Reference In"=w221, "error in"=w222, "Read(T)/Write(F)"=FALSE) -> ("FPGA VI Reference Out"=w223:refnum<k20>)  [unwired: 1 out]
            n112 = Number To Boolean Array(number=w229) -> (Boolean array=w231:bool[])
            n113 = Reverse 1D Array(array=w231) -> (reversed array=w232:bool[])
            n114 = Build Array (concatenate)(w230, w232) -> (w227:bool[])
            n115 = xnode "Read/Write Control"("FPGA VI Reference In"=w223, "Write Data"=w227) -> ("FPGA VI Reference Out"=w219:refnum<k20>)  [unwired: 1 in, 1 out]
            n116 = flat-sequence {
              tunnel: w219 -> [w242]
              tunnel: [w240] -> w220
              frame #0 {
                n117 = xnode "Read/Write Control"("FPGA VI Reference In"=w242, "Конфигурация"=TRUE) -> ("FPGA VI Reference Out"=w240:refnum<k20>)  [unwired: 1 in, 1 out]
                n118 = Wait (ms)(milliseconds to wait=u32 10) -> ()  [unwired: 1 out]
              }
            }
            n119 = flat-sequence {
              tunnel: w220 -> [w238]
              tunnel: [w236] -> _
              frame #0 {
                n120 = xnode "Read/Write Control"("FPGA VI Reference In"=w238, "Конфигурация"=FALSE) -> ("FPGA VI Reference Out"=w236:refnum<k20>)  [unwired: 1 in, 1 out]
                n121 = Wait (ms)(milliseconds to wait=u32 10) -> ()  [unwired: 1 out]
              }
            }
          }
          frame #5 {
            w253 = FALSE
            # "GREEN PGA"
            n122 = Decrement(x="Усиление (до 6)_GREEN") -> (x-1=w245:u8)
            n123 = Multiply(x=w245, y=378) -> (x*y=w247:i32)
            n124 = Multiply(x="Усиление (до 6)_GREEN", y=5) -> (x*y=w250:i32)
            n125 = xnode "Read/Write Control"("FPGA VI Reference In"=w258, "Enum"=T4."GREEN PGA" ("PGA")) -> ("FPGA VI Reference Out"=w256:refnum<k20>)  [unwired: 1 in, 1 out]
            n126 = Divide(x=w247, y=w250) -> (x/y=w251:dbl)
            n127 = Number To Boolean Array(number=w251) -> (Boolean array=w244:bool[])
            n128 = xnode "Read/Write Control"("FPGA VI Reference In"=w256, "Read(T)/Write(F)"=FALSE) -> ("FPGA VI Reference Out"=w255:refnum<k20>)  [unwired: 1 in, 1 out]
            n129 = Build Array (concatenate)(w253, w253, w253, w244) -> (w252:bool[])
            n130 = xnode "Read/Write Control"("FPGA VI Reference In"=w255, "Write Data"=w252) -> ("FPGA VI Reference Out"=w257:refnum<k20>)  [unwired: 1 in, 1 out]
            n131 = flat-sequence {
              tunnel: [w266] -> w259
              tunnel: w257 -> [w265]
              frame #0 {
                n132 = xnode "Read/Write Control"("FPGA VI Reference In"=w265, "Конфигурация"=TRUE) -> ("FPGA VI Reference Out"=w266:refnum<k20>)  [unwired: 1 in, 1 out]
                n133 = Wait (ms)(milliseconds to wait=u32 10) -> ()  [unwired: 1 out]
              }
            }
            n134 = flat-sequence {
              tunnel: w259 -> [w263]
              tunnel: [w261] -> _
              frame #0 {
                n135 = xnode "Read/Write Control"("FPGA VI Reference In"=w263, "Конфигурация"=FALSE) -> ("FPGA VI Reference Out"=w261:refnum<k20>)  [unwired: 1 in, 1 out]
                n136 = Wait (ms)(milliseconds to wait=u32 10) -> ()  [unwired: 1 out]
              }
            }
          }
          frame #6 {
            w271 = FALSE
            # "BLUE PGA"
            n137 = Decrement(x="Усиление (до 6)_BLUE") -> (x-1=w275:u8)
            n138 = Multiply(x=w275, y=378) -> (x*y=w276:i32)
            n139 = Multiply(x="Усиление (до 6)_BLUE", y=5) -> (x*y=w278:i32)
            n140 = xnode "Read/Write Control"("FPGA VI Reference In"=w268, "Enum"=T4."BLUE PGA" ("PGA")) -> ("FPGA VI Reference Out"=w282:refnum<k20>)  [unwired: 1 in, 1 out]
            n141 = Divide(x=w276, y=w278) -> (x/y=w279:dbl)
            n142 = Number To Boolean Array(number=w279) -> (Boolean array=w274:bool[])
            n143 = xnode "Read/Write Control"("FPGA VI Reference In"=w282, "Read(T)/Write(F)"=FALSE) -> ("FPGA VI Reference Out"=w281:refnum<k20>)  [unwired: 1 in, 1 out]
            n144 = Build Array (concatenate)(w271, w271, w271, w274) -> (w280:bool[])
            n145 = xnode "Read/Write Control"("FPGA VI Reference In"=w281, "Write Data"=w280) -> ("FPGA VI Reference Out"=w283:refnum<k20>)  [unwired: 1 in, 1 out]
            n146 = flat-sequence {
              tunnel: [w291] -> w284
              tunnel: w283 -> [w290]
              frame #0 {
                n147 = xnode "Read/Write Control"("FPGA VI Reference In"=w290, "Конфигурация"=TRUE) -> ("FPGA VI Reference Out"=w291:refnum<k20>)  [unwired: 1 in, 1 out]
                n148 = Wait (ms)(milliseconds to wait=u32 10) -> ()  [unwired: 1 out]
              }
            }
            n149 = flat-sequence {
              tunnel: w284 -> [w288]
              tunnel: [w286] -> _
              frame #0 {
                n150 = xnode "Read/Write Control"("FPGA VI Reference In"=w288, "Конфигурация"=FALSE) -> ("FPGA VI Reference Out"=w286:refnum<k20>)  [unwired: 1 in, 1 out]
                n151 = Wait (ms)(milliseconds to wait=u32 10) -> ()  [unwired: 1 out]
              }
            }
          }
          frame #7 {
            w304 = FALSE
            # "RED PGA"
            n152 = Decrement(x="Усиление (до 6)_RED") -> (x-1=w296:u8)
            n153 = Multiply(x=w296, y=378) -> (x*y=w298:i32)
            n154 = Multiply(x="Усиление (до 6)_RED", y=5) -> (x*y=w301:i32)
            n155 = xnode "Read/Write Control"("FPGA VI Reference In"=w293, "Enum"=T4."RED PGA" ("PGA")) -> ("FPGA VI Reference Out"=w307:refnum<k20>)  [unwired: 1 in, 1 out]
            n156 = Divide(x=w298, y=w301) -> (x/y=w302:dbl)
            n157 = Number To Boolean Array(number=w302) -> (Boolean array=w295:bool[])
            n158 = xnode "Read/Write Control"("FPGA VI Reference In"=w307, "Read(T)/Write(F)"=FALSE) -> ("FPGA VI Reference Out"=w306:refnum<k20>)  [unwired: 1 in, 1 out]
            n159 = Build Array (concatenate)(w304, w304, w304, w295) -> (w303:bool[])
            n160 = xnode "Read/Write Control"("FPGA VI Reference In"=w306, "Write Data"=w303) -> ("FPGA VI Reference Out"=w308:refnum<k20>)  [unwired: 1 in, 1 out]
            n161 = flat-sequence {
              tunnel: [w316] -> w309
              tunnel: w308 -> [w315]
              frame #0 {
                n162 = xnode "Read/Write Control"("FPGA VI Reference In"=w315, "Конфигурация"=TRUE) -> ("FPGA VI Reference Out"=w316:refnum<k20>)  [unwired: 1 in, 1 out]
                n163 = Wait (ms)(milliseconds to wait=u32 10) -> ()  [unwired: 1 out]
              }
            }
            n164 = flat-sequence {
              tunnel: w309 -> [w313]
              tunnel: [w311] -> _
              frame #0 {
                n165 = xnode "Read/Write Control"("FPGA VI Reference In"=w313, "Конфигурация"=FALSE) -> ("FPGA VI Reference Out"=w311:refnum<k20>)  [unwired: 1 in, 1 out]
                n166 = Wait (ms)(milliseconds to wait=u32 10) -> ()  [unwired: 1 out]
              }
            }
          }
          frame #8 {
            # "MUX"
            n167 = xnode "Read/Write Control"("FPGA VI Reference In"=w326, "Enum"=T4."MUX") -> ("FPGA VI Reference Out"=w320:refnum<k20>)  [unwired: 1 in, 1 out]
            n168 = case shown="\"GREEN\"" "Какой канал?" {
              tunnel: [bool[] [FALSE, TRUE, FALSE, TRUE, FALSE, FALSE, FALSE, FALSE, FALSE] ("MUX_register") bool[] [FALSE, TRUE, TRUE, FALSE, FALSE, FALSE, FALSE, FALSE, FALSE] ("MUX_register") bool[] [FALSE, TRUE, FALSE, FALSE, TRUE, FALSE, FALSE, FALSE, FALSE] ("MUX_register")] -> w318
              frame "GREEN" {
              }
              frame "RED", Default {
              }
              frame "BLUE" {
              }
            }
            n169 = xnode "Read/Write Control"("FPGA VI Reference In"=w320, "Read(T)/Write(F)"=FALSE) -> ("FPGA VI Reference Out"=w322:refnum<k20>)  [unwired: 1 in, 1 out]
            n170 = xnode "Read/Write Control"("FPGA VI Reference In"=w322, "Write Data"=w318) -> ("FPGA VI Reference Out"=w323:refnum<k20>)  [unwired: 1 in, 1 out]
            n171 = flat-sequence {
              tunnel: [w336] -> w324
              tunnel: w323 -> [w335]
              frame #0 {
                n172 = xnode "Read/Write Control"("FPGA VI Reference In"=w335, "Конфигурация"=TRUE) -> ("FPGA VI Reference Out"=w336:refnum<k20>)  [unwired: 1 in, 1 out]
                n173 = Wait (ms)(milliseconds to wait=u32 10) -> ()  [unwired: 1 out]
              }
            }
            n174 = flat-sequence {
              tunnel: w324 -> [w333]
              tunnel: [w331] -> _
              frame #0 {
                n175 = xnode "Read/Write Control"("FPGA VI Reference In"=w333, "Конфигурация"=FALSE) -> ("FPGA VI Reference Out"=w331:refnum<k20>)  [unwired: 1 in, 1 out]
                n176 = Wait (ms)(milliseconds to wait=u32 10) -> ()  [unwired: 1 out]
              }
            }
          }
          frame #9 {
            "АЦП прошит!" <- TRUE ("АЦП прошит!")
          }
        }
      }
    }
    n177 = local read "Стоп"() -> (w102:bool)
  }
  n178 = while {
    tunnel: w1 -> [w341]
    shift-right: [w340] -> _
    shift-left: _ -> [w339]
    stop <- w343 stop-if-true
    n179 = local read "Запись в FIFO"() -> (w342:bool)
    n180 = case shown="True" w342 {
      tunnel: [w346 w350] -> w343
      tunnel: w341 -> [_ w349]
      tunnel: [w345 w348] -> w340
      tunnel: w339 -> [w345 _]
      frame False {
        n181 = Wait (ms)(milliseconds to wait=u32 1) -> ()  [unwired: 1 out]
        n182 = local read "Стоп"() -> (w346:bool)
      }
      frame True {
        n183 = flat-sequence {
          tunnel: w349 -> [w354]
          tunnel: [w352] -> w347
          tunnel: [w387] -> w350
          tunnel: [w386] -> w348
          tunnel: w347 -> [w386]
          frame #0 {
            w357 = T5 6 items=["Grayscale (U8)", "Grayscale (I16)", "Grayscale (SGL)", "Complex (CSG)", "RGB (U32)", "HSL (U32)", "RGB (U64)"] ("Image Type")
            # "L"
            # "H"
            n184 = xnode "Invoke Method"("FPGA VI Reference In"=w354, "Number of Elements"=u32 4174, "Timeout (ms)"=2000) -> ("Data"=w361:u8[])  [unwired: 1 in, 3 out]
            n185 = Wait (ms)(milliseconds to wait="Кадр виден?") -> ()  [unwired: 1 out]
            n186 = Decimate 1D Array(w361) -> (w362:u8[], w363:u8[])
            n187 = for {
              N: 2087 -> [_]
              tunnel: w362 -> [w385]
              tunnel: w363 -> [w384]
              tunnel: [w376] -> w353 mode=indexing
              i -> [w383]
              n188 = Index Array(array=w384, index=w383) -> (element=w381:u8)
              n189 = Index Array(array=w385, index=w383) -> (element=w382:u8)
              n190 = To Unsigned Word Integer(number=w382) -> (unsigned 16bit integer=w380:u16)
              n191 = To Unsigned Word Integer(number=w381) -> (unsigned 16bit integer=w377:u16)
              n192 = Multiply(x=w380, y=u16 256) -> (x*y=w378:u16)
              n193 = Add(x=w378, y=w377) -> (x+y=w376:u16)
            }
            n194 = for {
              N: 58 -> [_]
              tunnel: [w369] -> w355 mode=indexing
              shift-right: [w368] -> _
              shift-left: w353 -> [w371]
              n195 = Delete From Array(array=w371, length=36, index=0) -> (deleted portion=w369:u16[], array with subset deleted=w368:u16[])
            }
            "DATA" <- w355
            n196 = for {
              tunnel: w355 -> [w373] mode=indexing
              tunnel: [w372] -> w360 mode=indexing
              n197 = for {
                tunnel: [w375] -> w372 mode=indexing
                tunnel: w373 -> [w374] mode=indexing
                n198 = Bundle(w374, w374, w374, w374) -> (w375:cluster{u16, u16, u16, u16})  [unwired: 1 in]
              }
            }
            n199 = call "IMAQ Create"("Image Name"="ILX751B", "Image Type"=w357) -> ("New Image"=w359:T1)  [unwired: 3 in, 1 out]
            n200 = call "IMAQ ArrayToColorImage"("Image"=w359, "Image Pixels (U64)"=w360) -> ("Image Out"=w352:T1)  [unwired: 3 in, 1 out]
          }
          frame #1 {
            n201 = local read "Стоп"() -> (w387:bool)
          }
        }
      }
    }
    "Image" <- w340
  }
  n202 = while {
    tunnel: w10 -> [w396]
    tunnel: w9 -> [w395]
    tunnel: w8 -> [_]
    shift-right: [w393] -> _
    shift-left: FALSE ("Питание") -> [w394]
    tunnel: [w391] -> w7
    tunnel: [w390] -> w6
    tunnel: w2 -> [w388]
    stop <- w392 stop-if-true
    n203 = Wait (ms)(milliseconds to wait=u32 1) -> ()  [unwired: 1 out]
    n204 = stacked-sequence {
      tunnel: w396 -> [w406 w440 w492]
      tunnel: w395 -> [w405 w439 w491]
      tunnel: w394 -> [_ w444 _]
      tunnel: [_ "Питание" _] -> w393
      tunnel: [_ "Стоп" _] -> w392
      tunnel: [_ _ w492] -> w391
      tunnel: [_ _ w491] -> w390
      tunnel: w388 -> [w403 w438 _]
      frame #0 {
        w397 = T6 0 items=["Current", "Voltage"] ("measurement type")
        n205 = call <instrlib>:"niDCPower Configure Current Limit.vi"("current limit"="A_POW_curlim", "channel name"="0", "instrument handle"=w406) -> ("instrument handle out"=w431:refnum<k15>)  [unwired: 7 in, 1 out]
        n206 = call <instrlib>:"niDCPower Configure Current Limit.vi"("current limit"="VDD1(9)_curlim", "channel name"="1", "instrument handle"=w406) -> ("instrument handle out"=w432:refnum<k15>)  [unwired: 7 in, 1 out]
        n207 = call <instrlib>:"niDCPower Configure Current Limit.vi"("current limit"="D_POW_curlim", "channel name"="0", "instrument handle"=w405) -> ("instrument handle out"=w415:refnum<k15>)  [unwired: 7 in, 1 out]
        n208 = call <instrlib>:"niDCPower Configure Current Limit.vi"("current limit"="VDD2(5)_curlim", "channel name"="1", "instrument handle"=w405) -> ("instrument handle out"=w416:refnum<k15>)  [unwired: 7 in, 1 out]
        n209 = call <instrlib>:"niDCPower Configure Current Limit.vi"("current limit"=0.1, "channel name"="0", "instrument handle"=w403) -> ("instrument handle out"=w402:refnum<k15>)  [unwired: 7 in, 1 out]
        n210 = call <instrlib>:"niDCPower Configure Voltage Level.vi"("voltage level"="A_POW, V", "channel name"="0", "instrument handle"=w431) -> ("instrument handle out"=w425:refnum<k15>)  [unwired: 7 in, 1 out]
        n211 = call <instrlib>:"niDCPower Configure Voltage Level.vi"("voltage level"="VDD1(9), V", "channel name"="1", "instrument handle"=w432) -> ("instrument handle out"=w424:refnum<k15>)  [unwired: 7 in, 1 out]
        n212 = call <instrlib>:"niDCPower Configure Voltage Level.vi"("voltage level"="D_POW, V", "channel name"="0", "instrument handle"=w415) -> ("instrument handle out"=w410:refnum<k15>)  [unwired: 7 in, 1 out]
        n213 = call <instrlib>:"niDCPower Configure Voltage Level.vi"("voltage level"="VDD2(5), V", "channel name"="1", "instrument handle"=w416) -> ("instrument handle out"=w409:refnum<k15>)  [unwired: 7 in, 1 out]
        n214 = call <instrlib>:"niDCPower Configure Voltage Level.vi"("voltage level"=5.0, "channel name"="0", "instrument handle"=w402) -> ()  [unwired: 7 in, 2 out]
        n215 = call <instrlib>:"niDCPower Measure.vi"("measurement type"=w397, "channel name"="0", "instrument handle"=w425) -> ("measurement"=→"A_POW_cur" →"A_POW_char":dbl)  [unwired: 6 in, 2 out]
        n216 = call <instrlib>:"niDCPower Measure.vi"("measurement type"=w397, "channel name"="0", "instrument handle"=w410) -> ("measurement"=→"D_POW_cur" →"D_POW_char":dbl)  [unwired: 6 in, 2 out]
        n217 = call <instrlib>:"niDCPower Measure.vi"("measurement type"=w397, "channel name"="1", "instrument handle"=w424) -> ("measurement"=→"VDD1(9)_cur" →"VDD1(9)_char":dbl)  [unwired: 6 in, 2 out]
        n218 = call <instrlib>:"niDCPower Measure.vi"("measurement type"=w397, "channel name"="1", "instrument handle"=w409) -> ("measurement"=→"VDD2(5)_cur" →"VDD2(5)_char":dbl)  [unwired: 6 in, 2 out]
      }
      frame #1 {
        n219 = Less?(x="Питание", y=w444) -> (x < y?=w443:bool)
        n220 = Not(x="Стоп") -> (.not. x?=w446:bool)
        n221 = Greater?(x="Питание", y=w444) -> (0:w447:bool)
        n222 = Or(x="Стоп", y=w443) -> (x .or. y?=w441:bool)
        n223 = And(x=w446, y=w447) -> (x .and. y?=w448:bool)
        n224 = case shown="True" w448 {
          tunnel: w440 -> [_ w474]
          tunnel: w439 -> [_ w473]
          tunnel: w438 -> [_ w468]
          frame False {
          }
          frame True {
            # "Включение"
            n225 = flat-sequence {
              tunnel: w474 -> [w479]
              tunnel: w473 -> [w478]
              tunnel: [w479] -> w471
              tunnel: [w478] -> w469
              tunnel: w468 -> [w477]
              tunnel: [w483] -> w472
              tunnel: w471 -> [w483]
              tunnel: [w482] -> w470
              tunnel: w469 -> [w482]
              tunnel: w472 -> [w486]
              tunnel: w470 -> [w485]
              frame #0 {
                # "VDD1"
                n226 = call <instrlib>:"niDCPower Configure Output Enabled.vi"("output enabled"=TRUE, "channel name"="1", "instrument handle"=w479) -> ()  [unwired: 7 in, 2 out]
                n227 = call <instrlib>:"niDCPower Configure Output Enabled.vi"("output enabled"=TRUE, "channel name"="0", "instrument handle"=w477) -> ()  [unwired: 7 in, 2 out]
              }
              frame #1 {
                n228 = Wait (ms)(milliseconds to wait=u32 50) -> ()  [unwired: 1 out]
              }
              frame #2 {
                # "D_POW+VDD2"
                # "A_POW"
                n229 = call <instrlib>:"niDCPower Configure Output Enabled.vi"("output enabled"=TRUE, "channel name"="0", "instrument handle"=w486) -> ()  [unwired: 7 in, 2 out]
                n230 = call <instrlib>:"niDCPower Configure Output Enabled.vi"("output enabled"=TRUE, "channel name"="0,1", "instrument handle"=w485) -> ()  [unwired: 7 in, 2 out]
              }
            }
          }
        }
        n231 = case shown="True" w441 {
          tunnel: w440 -> [_ w453]
          tunnel: w439 -> [_ w452]
          tunnel: w438 -> [_ w449]
          frame False {
          }
          frame True {
            # "A_POW"
            # "Выключение"
            n232 = flat-sequence {
              tunnel: w453 -> [w457]
              tunnel: w452 -> [w458]
              tunnel: [w457] -> w450
              tunnel: w449 -> [w454]
              tunnel: [w463] -> w451
              tunnel: w450 -> [w463]
              tunnel: w451 -> [w465]
              frame #0 {
                # "D_POW+VDD2"
                n233 = call <instrlib>:"niDCPower Configure Output Enabled.vi"("output enabled"=FALSE, "channel name"="0", "instrument handle"=w457) -> ()  [unwired: 7 in, 2 out]
                n234 = call <instrlib>:"niDCPower Configure Output Enabled.vi"("output enabled"=FALSE, "channel name"="0", "instrument handle"=w454) -> ()  [unwired: 7 in, 2 out]
                n235 = call <instrlib>:"niDCPower Configure Output Enabled.vi"("output enabled"=FALSE, "channel name"="0,1", "instrument handle"=w458) -> ()  [unwired: 7 in, 2 out]
              }
              frame #1 {
                n236 = Wait (ms)(milliseconds to wait=u32 50) -> ()  [unwired: 1 out]
              }
              frame #2 {
                # "VDD1"
                n237 = call <instrlib>:"niDCPower Configure Output Enabled.vi"("output enabled"=FALSE, "channel name"="1", "instrument handle"=w465) -> ()  [unwired: 7 in, 2 out]
              }
            }
          }
        }
      }
      frame #2 {
      }
    }
  }
  n238 = while {
    tunnel: w1 -> [w496]
    tunnel: w1 -> [w494]
    tunnel: w1 -> [w493]
    stop <- w497 stop-if-true
    n239 = flat-sequence {
      tunnel: w496 -> [w529]
      tunnel: w494 -> [w501]
      tunnel: w493 -> [w499]
      tunnel: [w530] -> w497
      frame #0 {
        n240 = local read "Стоп"() -> (w527:bool)
        n241 = local read "Питание"() -> (w524:bool)
        n242 = xnode "Read/Write Control"("FPGA VI Reference In"=w501, "Задержка, мкс"="Задержка, мкс") -> ()  [unwired: 1 in, 2 out]
        n243 = Not(x=w527) -> (.not. x?=w526:bool)
        n244 = xnode "Read/Write Control"("FPGA VI Reference In"=w499, "8191?"="8191?") -> ()  [unwired: 1 in, 2 out]
        n245 = Add(x=u16 40, y="SHUT1") -> (x+y=w503:u16)
        n246 = Compound Arithmetic op=AND(w526, "Линейки", w524) -> (w523:bool)
        n247 = xnode "Read/Write Control"("FPGA VI Reference In"=w529, "Запись в FIFO"="Запись в FIFO", "Направление бит"="Направление бит", "Остановка основного цикла"=w527, "Линейки"=w523, "CDS1_1"="CDS1_1", "CDS1_2"="CDS1_2", "CDS2_1"="CDS2_1", "CDS2_2"="CDS2_2", "ADC_1"="ADC_1", "ADC_2"="ADC_2", "П_41789?"="П_41789?", "42000?"="42000?", "20"="20", "CLK_3"="CLK_3", "CLK_2"="CLK_2", "SHUT_2"=w503, "SHUT1"="SHUT1", "ROG_2"="ROG_2", "ROG_1"="ROG_1", "CLK_1"="CLK_1", "LOW"="LOW", "HIGH"="HIGH", "50?"="50?") -> ()  [unwired: 1 in, 2 out]
      }
      frame #1 {
        n248 = local read "Стоп"() -> (w530:bool)
      }
    }
    n249 = Wait (ms)(milliseconds to wait=u32 25) -> ()  [unwired: 1 out]
  }
  n250 = while {
    tunnel: w4 -> [w538]
    stop <- w531 stop-if-true
    w545 = i16 3 ("width (-)")
    n251 = local read "A_POW_cur"() -> (w542:dbl)
    n252 = local read "VDD1(9)_cur"() -> (w541:dbl)
    n253 = local read "D_POW_cur"() -> (w540:dbl)
    n254 = local read "VDD2(5)_cur"() -> (w539:dbl)
    n255 = Get Date/Time In Seconds() -> (seconds since 1Jan1904=w547:timestamp)
    n256 = Format Date/Time String(time format string (%c)="%d %H:%M:%S:%3u", seconds (now)=w547) -> (date/time string=w544:string)  [unwired: 1 in]
    n257 = Number To Fractional String(number=w542, width (-)=w545, precision (6)=w545) -> (F-format string=w536:string)  [unwired: 1 in]
    n258 = Number To Fractional String(number=w541, width (-)=w545, precision (6)=w545) -> (F-format string=w535:string)  [unwired: 1 in]
    n259 = Number To Fractional String(number=w540, width (-)=w545, precision (6)=w545) -> (F-format string=w534:string)  [unwired: 1 in]
    n260 = Number To Fractional String(number=w539, width (-)=w545, precision (6)=w545) -> (F-format string=w533:string)  [unwired: 1 in]
    n261 = Concatenate Strings(w544, w536, w535, w534, w533, "\t") -> (w537:string)
    n262 = Format Into String(initial string=w538, w537) -> ()  [unwired: 2 in, 2 out]
    n263 = Wait (ms)(milliseconds to wait=u32 2000) -> ()  [unwired: 1 out]
    n264 = local read "Стоп"() -> (w531:bool)
  }
  n265 = while {
    shift-right: [w552] -> _
    shift-left: _ -> [w553]
    tunnel: w3 -> [w549]
    tunnel: w4 -> [_]
    stop <- w554 stop-if-true
    n266 = local read "Питание"() -> (w552:bool)
    n267 = Wait (ms)(milliseconds to wait=u32 1) -> ()  [unwired: 1 out]
    n268 = flat-sequence {
      tunnel: w551 -> [w556]
      tunnel: [w555] -> w550
      tunnel: w549 -> [w555]
      tunnel: w550 -> [w558]
      frame #0 {
        n269 = case shown="True" w556 {
          frame False {
          }
          frame True {
            n270 = Wait (ms)(milliseconds to wait=u32 100) -> ()  [unwired: 1 out]
          }
        }
      }
      frame #1 {
        n271 = local read "A_POW_cur"() -> (w571:dbl)
        n272 = local read "VDD1(9)_cur"() -> (w569:dbl)
        n273 = local read "D_POW_cur"() -> (w567:dbl)
        n274 = local read "VDD2(5)_cur"() -> (w565:dbl)
        n275 = Greater Or Equal?(x=w567, y="D_POW_selcur") -> (x >= y?=w561:bool)
        "D_POW" <- w561
        n276 = Greater Or Equal?(x=w569, y="VDD1(9)_selcur") -> (x >= y?=w562:bool)
        "VDD1(9)" <- w562
        n277 = Greater Or Equal?(x=w565, y="VDD2(5)_selcur") -> (x >= y?=w560:bool)
        "VDD2(5)" <- w560
        n278 = Greater Or Equal?(x=w571, y="A_POW_selcur") -> (x >= y?=w563:bool)
        "A_POW" <- w563
        n279 = Compound Arithmetic op=OR(w563, w562, w561, w560) -> (w559:bool)
        n280 = case shown="True" w559 {
          tunnel: w558 -> [_ w573]
          frame False {
          }
          frame True {
            n281 = local write "Запись кадра"(FALSE ("Запись кадра")) -> ()
            n282 = local write "Питание"(FALSE) -> ()
            n283 = xnode "Read/Write Control"("FPGA VI Reference In"=w573, "Линейки"=FALSE) -> ()  [unwired: 1 in, 2 out]
          }
        }
      }
    }
    n284 = Greater?(x=w552, y=w553) -> (0:w551:bool)
    n285 = local read "Стоп"() -> (w554:bool)
  }
  n286 = while {
    shift-right: ["Запись кадра"] -> _
    shift-left: _ -> [w593]
    tunnel: w1 -> [_]
    stop <- w594 stop-if-true
    n287 = local read "Задержка, мкс"() -> (w578:u16)
    n288 = local read "SHUT1"() -> (w589:u16)
    n289 = local read "42000?"() -> (w586:u16)
    n290 = local read "ROG_2"() -> (w588:u16)
    n291 = Subtract(x=w589, y=w588) -> (x-y=w587:u16)
    n292 = Greater?(x="Запись кадра", y=w593) -> (0:w591:bool)
    n293 = Subtract(x=w586, y=w587) -> (x-y=w582:u16)
    n294 = To Double Precision Float(number=w578) -> (double precision float=w577:dbl)
    n295 = To Double Precision Float(number=w582) -> (double precision float=w581:dbl)
    n296 = Divide(x=w577, y=1000.0 ("x")) -> (x/y=w584:dbl)
    n297 = Multiply(x=w581, y=50.0) -> (x*y=w580:dbl)
    n298 = Divide(x=w580, y=1000000.0) -> (x/y=w585:dbl)
    n299 = Add(x=w585, y=w584) -> (x+y=w583:dbl)
    "Тнак, мс" <- w583
    n300 = case shown="True" w591 {
      tunnel: w583 -> [_ w596]
      frame False {
        n301 = Wait (ms)(milliseconds to wait=u32 10) -> ()  [unwired: 1 out]
      }
      frame True {
        w598 = i16 0 ("width (-)")
        w610 = "_"
        n302 = local read "Номер образца"() -> (w601:string)
        n303 = local read "Температура"() -> (w604:string)
        n304 = Concatenate Strings("Темп. = " ("string"), w604) -> (w602:string)
        n305 = Get Date/Time In Seconds() -> (seconds since 1Jan1904=w626:timestamp)
        n306 = Concatenate Strings("Образец_" ("string"), w601) -> (w599:string)
        n307 = Number To Fractional String(number=w596, width (-)=w598, precision (6)=w598) -> (F-format string=w611:string)  [unwired: 1 in]
        n308 = Format Date/Time String(time format string (%c)="%H.%M.%S", seconds (now)=w626) -> (date/time string=w630:string)  [unwired: 1 in]
        n309 = Select(t="Светло", s="Светлый (T)\nТемный (F)", f="Темно") -> (s? t:f=w627:string)
        n310 = Build Path(base path="Frames", name or relative path=w599) -> (appended path=w621:path)
        n311 = call <vilib>:"Check if File or Folder Exists.vi"("path"=w621) -> ("file or folder exists?"=w620:bool, "dup path"=w619:path)  [unwired: 8 in, 1 out]
        n312 = local read "Image"() -> (w613:T1)
        n313 = Concatenate Strings(w630, w610, "ПРИМЕЧАНИЕ", w610, "Тн(мс)=" ("string"), w611, ".tiff" ("element")) -> (w629:string)
        n314 = case shown="False" w620 {
          tunnel: w619 -> [w639 w640]
          tunnel: [w638 w640] -> w606
          frame False {
            n315 = Create Folder(path (use dialog)=w639) -> (created path=w638:path)  [unwired: 2 in, 2 out]
          }
          frame True {
          }
        }
        n316 = Build Path(base path=w606, name or relative path=w602) -> (appended path=w607:path)
        n317 = call <vilib>:"Check if File or Folder Exists.vi"("path"=w607) -> ("file or folder exists?"=w608:bool, "dup path"=w609:path)  [unwired: 8 in, 1 out]
        n318 = case shown="False" w608 {
          tunnel: w609 -> [w633 w634]
          tunnel: [w632 w634] -> w605
          frame False {
            n319 = Create Folder(path (use dialog)=w633) -> (created path=w632:path)  [unwired: 2 in, 2 out]
          }
          frame True {
          }
        }
        n320 = Build Path(base path=w605, name or relative path=w627) -> (appended path=w622:path)
        n321 = call <vilib>:"Check if File or Folder Exists.vi"("path"=w622) -> ("file or folder exists?"=w623:bool, "dup path"=w624:path)  [unwired: 8 in, 1 out]
        n322 = case shown="False" w623 {
          tunnel: w624 -> [w636 w637]
          tunnel: [w635 w637] -> w628
          frame False {
            n323 = Create Folder(path (use dialog)=w636) -> (created path=w635:path)  [unwired: 2 in, 2 out]
          }
          frame True {
          }
        }
        n324 = Build Path(base path=w628, name or relative path=w629) -> (appended path=w625:path)
        n325 = call-poly "IMAQ Write File 2"("File Path"=w625, "Image"=w613) -> ()  [unwired: 8 in, 2 out]
      }
    }
    n326 = local read "Стоп"() -> (w594:bool)
  }
  n327 = while {
    tunnel: w1 -> [_]
    stop <- w678 stop-if-true
    n328 = local read "DATA"() -> (w679:u16[][])
    n329 = property on="Image" class="ImageControl"() -> ("ROI"=w680:T7)  [unwired: 2 in, 2 out]
    n330 = Unbundle By Name(w680) -> ("Contours"=w692:T8)
    n331 = Index Array(array=w692, index=0) -> (element=w690:T9)
    n332 = Unbundle By Name(w690) -> ("Points"=w689:i32[])
    n333 = Index Array(array=w689, index=0) -> (element=w683:i32)
    n334 = Index Array(array=w689, index=1) -> (element=w681:i32)
    n335 = Index Array(array=w689, index=2) -> (element=w684:i32)
    n336 = Index Array(array=w689, index=3) -> (element=w682:i32)
    n337 = Subtract(x=w684, y=w683) -> (x-y=w677:i32)
    n338 = Subtract(x=w682, y=w681) -> (x-y=w676:i32)
    n339 = for {
      N: w677 -> [_]
      tunnel: w683 -> [w713]
      tunnel: w681 -> [w710]
      tunnel: w676 -> [w709]
      tunnel: w679 -> [w712]
      tunnel: [w708] -> w663 mode=indexing
      i -> [w714]
      n340 = Add(x=w713, y=w714) -> (x+y=w707:i32)
      n341 = Index Array(array=w712, index (col)=w707) -> (element=w711:u16[])  [unwired: 1 in]
      n342 = Delete From Array(array=w711, length=w709, index=w710) -> (deleted portion=w708:u16[])  [unwired: 1 out]
    }
    n343 = local read "Стоп"() -> (w678:bool)
    n344 = Multiply(x=w677, y=w676) -> (x*y=w662:i32)
    n345 = Reshape Array(w663, w662) -> (w651:u16[])
    n346 = To Double Precision Float(number=w651) -> (double precision float=w649:dbl[])
    n347 = Wait (ms)(milliseconds to wait=u32 1000) -> ()  [unwired: 1 out]
    n348 = local read "2/4 V"() -> (w674:enum16{"2V", "4V"})
    n349 = case shown="\"2V\", Default" w674 {
      tunnel: [2000 4000] -> w643
      frame "2V", Default {
      }
      frame "4V" {
      }
    }
    n350 = Divide(x="Какой шум на других каналах, мВ?", y=w643) -> (x/y=w645:dbl)
    n351 = Multiply(x=w645, y=65536.0) -> (x*y=w642:dbl)
    n352 = for {
      tunnel: w649 -> [w695] mode=indexing
      tunnel: w642 -> [w694]
      tunnel: [w693] -> w648 mode=indexing
      n353 = Subtract(x=w695, y=w694) -> (x-y=w693:dbl)
    }
    n354 = Array Size(array=w648) -> (size(s)=w660:i32)
    n355 = Array Max & Min(array=w648) -> (max value=w672:dbl, min value=w671:dbl)  [unwired: 2 out]
    n356 = Array Size(array=w648) -> (size(s)=w658:i32)
    n357 = for {
      tunnel: w648 -> [w704] mode=indexing
      shift-right: [w702] -> w661
      shift-left: 0.0 -> [w703]
      n358 = Add(x=w704, y=w703) -> (x+y=w702:dbl)
    }
    n359 = Subtract(x=w672, y=w671) -> (x-y=w670:dbl)
    n360 = Divide(x=w661, y=w660) -> (x/y=w641:dbl)
    n361 = for {
      tunnel: w648 -> [w701] mode=indexing
      shift-right: [w697] -> w659
      shift-left: 0.0 -> [w698]
      tunnel: w641 -> [w696]
      n362 = Subtract(x=w696, y=w701) -> (x-y=w700:dbl)
      n363 = Square(x=w700) -> (x^2=w699:dbl)
      n364 = Add(x=w699, y=w698) -> (x+y=w697:dbl)
    }
    n365 = Multiply(x=w641, y=2.0) -> (x*y=w668:dbl)
    n366 = Divide(x=w659, y=w658) -> (x/y=w657:dbl)
    n367 = Divide(x=w670, y=w668) -> (x/y=w669:dbl)
    n368 = Square Root(x=w657) -> (sqrt(x)=w655:dbl)
    n369 = Divide(x=w641, y=65536.0) -> (x/y=w673:dbl)
    n370 = Multiply(x=w643, y=w673) -> (x*y=→"|Vout|, мВ":dbl)
    n371 = Divide(x=w655, y=65536.0) -> (x/y=w654:dbl)
    n372 = Multiply(x=w643, y=w654) -> (x*y=→"DSNU, мВ":dbl)
    n373 = Multiply(x=w669, y=100.0) -> (x*y=→"PRNU, %":dbl)
  }
  n374 = call <instrlib>:"niDCPower Close.vi"("instrument handle"=w7) -> ()  [unwired: 10 in, 1 out]
  n375 = call <instrlib>:"niDCPower Close.vi"("instrument handle"=w6) -> ()  [unwired: 10 in, 1 out]
